vi "Channels.vi"() -> (2 "Names":string[](array[string]), 3 "Channels to Create":T1[](array[typedef]) {"Custom Config Data" format="%x"})   [LabVIEW 2021, in "TemplateCommon.lvlib"]
uses:
  TemplateCommon.lvlib
  CIF-LVCore/src/Channels/ChannelRegistrar/typedef/Channel Definition.ctl
  <vilib>/CIF Foundation/CIF Channels Core/CIFChannels/Typedef/Direction.ctl
  CIF-LVCore/src/Channels/ChannelRegistrar/typedef/Registered Channel Types.ctl
  <vilib>/CIF Foundation/CIF Channels Core/ChannelCommon/Utilities/Flatten FIFO Config.vi
  <vilib>/CIF Foundation/CIF Channels Core/ChannelCommon/Utilities/Flatten FIFO Flags.vi
  <vilib>/CIF Foundation/CIF Utilities/DataTypes/Flatten Unflatten/Flatten U64.vi
  CIF-LVCore/src/Channels/ChannelRegistrar/ChannelRegistrar.lvlib
  <vilib>/CIF Foundation/CIF Channels Core/CIFChannels/CIFChannels.lvclass
  <vilib>/CIF Foundation/CIF Channels Core/ChannelCommon/ChannelCommon.lvlib
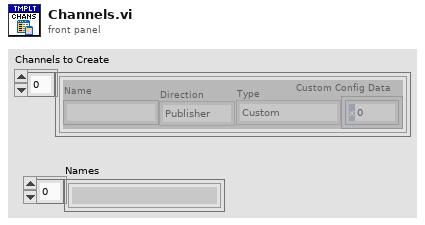
[diagram p1: front panel]
types:
  T1 = typedef "ChannelRegistrar.lvlib/Channel Definition.ctl" = cluster{"Name":string, "Direction":T2, "Type":T3, "Custom Config Data":u8[]}
  T2 = typedef "CIFChannels.lvclass/Direction.ctl" = enum16{"Publisher", "Subscriber"}
  T3 = typedef "ChannelRegistrar.lvlib/Registered Channel Types.ctl" = enum16{"Custom", "Double_Tag", "I64_Tag", "U64_Tag", "U8_FIFO", "CAN_FIFO", "L2Enet_FIFO", "DAQ_FIFO", "Universal_FIFO", "String_Tag"}
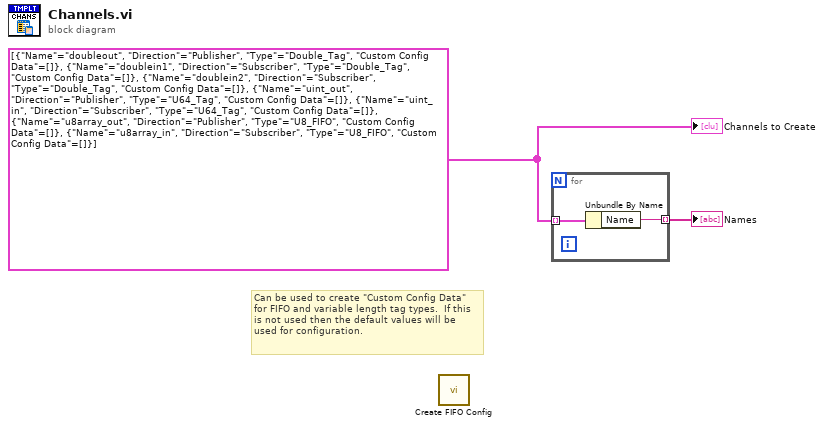
[diagram p0: block diagram]
diagram:
  w1 = T1[] [{"Name"="doubleout", "Direction"=enum."Publisher", "Type"=enum."Double_Tag", "Custom Config Data"=[]}, {"Name"="doublein1", "Direction"=enum."Subscriber", "Type"=enum."Double_Tag", "Custom Config Data"=[]}, {"Name"="doublein2", "Direction"=enum."Subscriber", "Type"=enum."Double_Tag", "Custom Config Data"=[]}, {"Name"="uint_out", "Direction"=enum."Publisher", "Type"=enum."U64_Tag", "Custom Config Data"=[]}, {"Name"="uint_in", "Direction"=enum."Subscriber", "Type"=enum."U64_Tag", "Custom Config Data"=[]}, {"Name"="u8array_out", "Direction"=enum."Publisher", "Type"=enum."U8_FIFO", "Custom Config Data"=[]}, {"Name"="u8array_in", "Direction"=enum."Subscriber", "Type"=enum."U8_FIFO", "Custom Config Data"=[]}] ("Channels to Create in")
  # "Can be used to create \"Custom Config Data\" for FIFO and variable length tag types.  If this is not used then the default values will be used for configuration."
  n1 = call <vilib>:"Create FIFO Config.vi"() -> ()  [unwired: 11 in, 1 out]
  n2 = for {
    tunnel: w1 -> [w4] mode=indexing
    tunnel: [w3] -> w2 mode=indexing
    n3 = Unbundle By Name(w4) -> ("Name"=w3:string)
  }
  "Names" <- w2
  "Channels to Create" <- w1
